vi "dsdll_capture_wave_variant.vi"(8 "error in":errorcluster, 10 "samples count in":u32, 11 "dsdll instance in":T2={"dsdll path"=path "E:/LVprog/DirectSoundDLL/dsdll.dll", "dsdll handle"=[], "output devices"=[], "capture devices"=[]}) -> (0 "error out":errorcluster, 1 "variant sample data":variant, 2 "samples count out":u32, 3 "dsdll instance out":T2, 4 "format":T1, 5 "time stamp [s]":dbl, 6 "channels count":u16)   [LabVIEW 2018, in "dsdll.lvlib"]
doc: "Call this to capture waveform of specified length.\nThis VI si synchronous so it won't return untill entire waveform is recorded.\n\nReturn format is variant that contains 2D array of samples in selected format where:\nrows = samples\ncolumns = channels"
uses:
  dsdll.lvlib
  dsdll_instance.ctl
  dsdll_device_record.ctl
  dsdll_sample_format.ctl
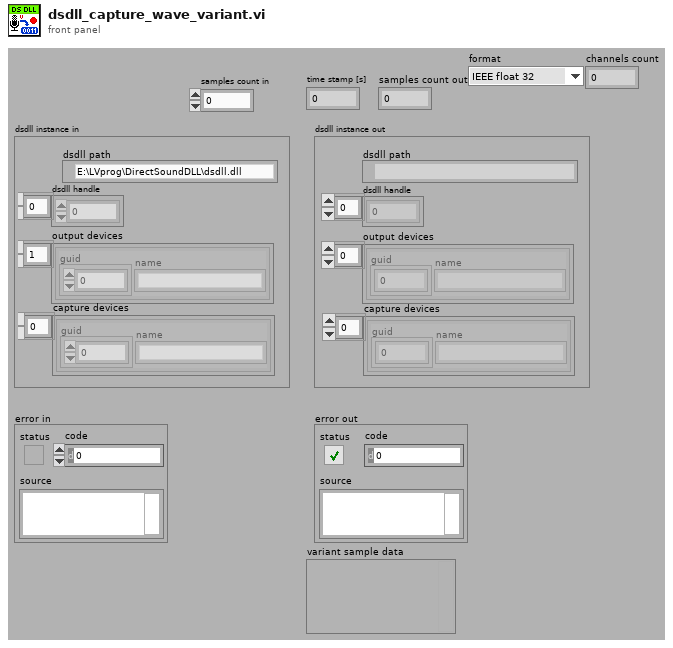
[diagram p1: front panel]
types:
  T1 = typedef "dsdll.lvlib/dsdll_sample_format.ctl" = enum16{"IEEE float 32", "PCM 16 bit"}
  T2 = typedef "dsdll.lvlib/dsdll_instance.ctl" = cluster{"dsdll path":path, "dsdll handle":u8[], "output devices":T3[], "capture devices":T3[]}
  T3 = typedef "dsdll.lvlib/dsdll_device_record.ctl" = cluster{"guid":u8[], "name":string}
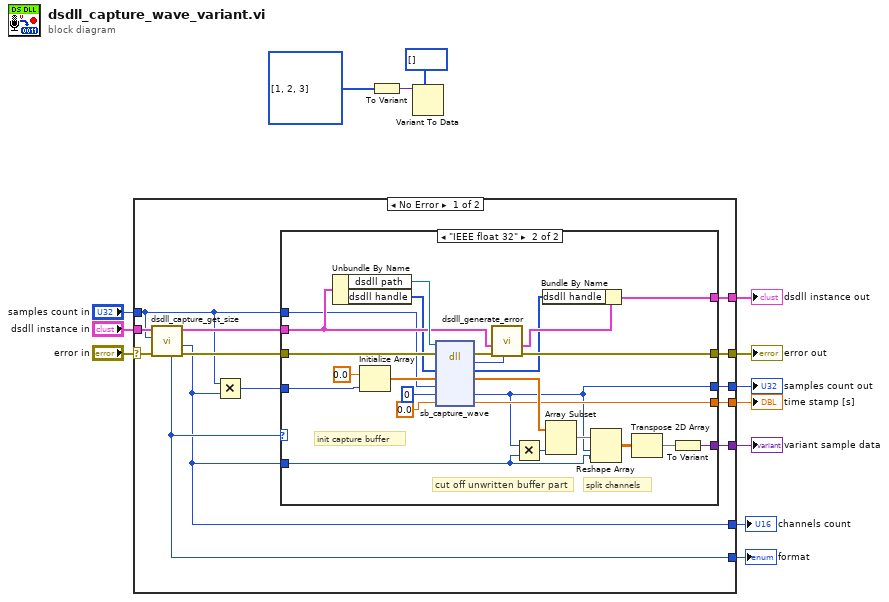
[diagram p0: block diagram]
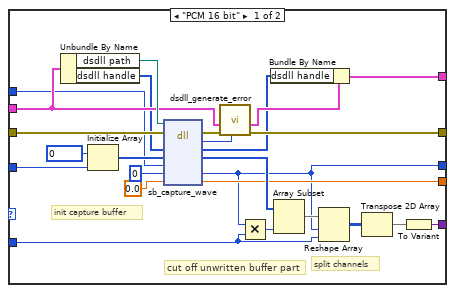
[diagram p2: hidden frame]
diagram:
  n1 = case shown="No Error" "error in" {
    selector: "error in" -> [w24 w77]
    tunnel: "dsdll instance in" -> [w23 w78]
    tunnel: [w26 w77] -> w12
    tunnel: [w25 w78] -> w13
    tunnel: "samples count in" -> [w16 _]
    tunnel: [w20 _] -> w8
    tunnel: [w19 _] -> w7
    tunnel: [w18 _] -> w3
    tunnel: [w17 _] -> w2
    tunnel: [w15 _] -> w1
    frame No Error {
      n2 = call "dsdll_capture_get_size.vi"("error in"=w24, "samples count"=w16, "dsdll instance in"=w23) -> ("error out"=w21:errorcluster, "channels count"=w15:u16, "dsdll instance out"=w22:T2, "format"=w17:T1)  [unwired: 3 in, 2 out]
      n3 = Multiply(x=w16, y=w15) -> (x*y=w14:u32)
      n4 = case shown="\"IEEE float 32\"" w17 {
        tunnel: [w49 w74] -> w26
        tunnel: [w46 w71] -> w25
        tunnel: w22 -> [w38 w64]
        tunnel: w21 -> [w37 w63]
        tunnel: w16 -> [w36 w62]
        tunnel: [w33 w59] -> w20
        tunnel: [w32 w58] -> w19
        tunnel: w15 -> [w29 w57]
        tunnel: [w31 w55] -> w18
        tunnel: w14 -> [w30 w53]
        frame "PCM 16 bit" {
          # "init capture buffer"
          # "split channels"
          # "cut off unwritten buffer part"
          n5 = Unbundle By Name(w38) -> ("dsdll path"=w40:path, "dsdll handle"=w35:u8[])
          n6 = Initialize Array(i16 0 ("bsize"), w30) -> (w44:i16[])
          n7 = dll-call lib="dsdll.dll" fn="sb_capture_wave" ("sb_get_handle_size()")(path in=w40, error in=w37, "handle"=w35, "data"=w44, "count"=w36, "read"=u32 0, "time_stamp"=0.0) -> (error out=w51:errorcluster, "error"=w50:i32, "handle"=w47:u8[], "data"=w41:i16[], "read"=w32:u32, "time_stamp"=w33:dbl)  [unwired: 2 in, 1 out]
          n8 = call "dsdll_generate_error.vi"("error code"=w50, "error in"=w51, "dsdll instance in"=w38) -> ("error out"=w49:errorcluster, "dsdll instance out"=w48:T2)  [unwired: 6 in, 1 out]
          n9 = Multiply(x=w32, y=w29) -> (x*y=w34:u32)
          n10 = Bundle By Name(cluster=w48, "dsdll handle"=w47) -> (w46:T2)
          n11 = Array Subset(array=w41, length=w34) -> (w39:i16[])  [unwired: 1 in]
          n12 = Reshape Array(w39, w32, w29) -> (w28:i16[][])
          n13 = Transpose 2D Array(2D array=w28) -> (transposed array=w27:i16[][])
          n14 = To Variant(anything=w27) -> (Variant=w31:variant)
        }
        frame "IEEE float 32" {
          # "init capture buffer"
          # "split channels"
          # "cut off unwritten buffer part"
          n15 = Unbundle By Name(w64) -> ("dsdll path"=w66:path, "dsdll handle"=w61:u8[])
          n16 = Initialize Array(sgl 0.0 ("element"), w53) -> (w70:sgl[])
          n17 = dll-call lib="dsdll.dll" fn="sb_capture_wave" ("sb_get_handle_size()")(path in=w66, error in=w63, "handle"=w61, "data"=w70, "count"=w62, "read"=u32 0, "time_stamp"=0.0) -> (error out=w76:errorcluster, "error"=w75:i32, "handle"=w72:u8[], "data"=w67:sgl[], "read"=w58:u32, "time_stamp"=w59:dbl)  [unwired: 2 in, 1 out]
          n18 = call "dsdll_generate_error.vi"("error code"=w75, "error in"=w76, "dsdll instance in"=w64) -> ("error out"=w74:errorcluster, "dsdll instance out"=w73:T2)  [unwired: 6 in, 1 out]
          n19 = Multiply(x=w58, y=w57) -> (x*y=w60:u32)
          n20 = Bundle By Name(cluster=w73, "dsdll handle"=w72) -> (w71:T2)
          n21 = Array Subset(array=w67, length=w60) -> (w65:sgl[])  [unwired: 1 in]
          n22 = Reshape Array(w65, w58, w57) -> (w56:sgl[][])
          n23 = Transpose 2D Array(2D array=w56) -> (transposed array=w52:sgl[][])
          n24 = To Variant(anything=w52) -> (Variant=w55:variant)
        }
      }
    }
    frame Error {
    }
  }
  "error out" <- w12
  "dsdll instance out" <- w13
  "time stamp [s]" <- w8
  "samples count out" <- w7
  "variant sample data" <- w3
  "format" <- w2
  "channels count" <- w1
  n25 = To Variant(anything=i16[] [1, 2, 3]) -> (Variant=w5:variant)
  n26 = Variant To Data(type=i16[] [], Variant=w5) -> ()  [unwired: 1 in, 2 out]
